vi "setHeaters.vi"(8 "error in":errorcluster, 10 "Heater2":bool, 11 "Heater1":bool) -> (0 "error out":errorcluster)   [LabVIEW 2024]
doc: "Funkcja służąca do sterowania 2 grzałkami w symulowanym piekarniku, numer wejścia odpowiada numerowi grzałki. Wartość TRUE wejścia włącza grzałkę, wartość FALSE wejścia wyłącza grzałkę."
uses:
  TypeDefs/Heater_interface.ctl
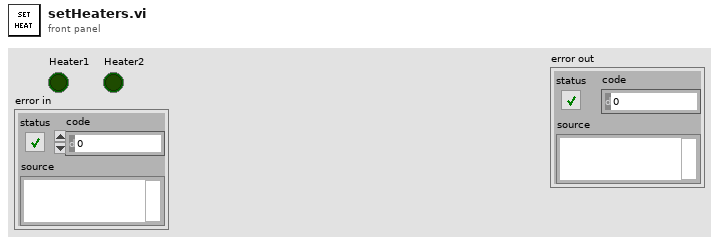
[diagram p1: front panel]
types:
  T1 = typedef "Heater_interface.ctl" = enum16{"setSpeed", "setHeaters", "getTemperature"}
  T2 = cluster{"Interface":T1, "Parameter1":variant, "Parameter2":variant}
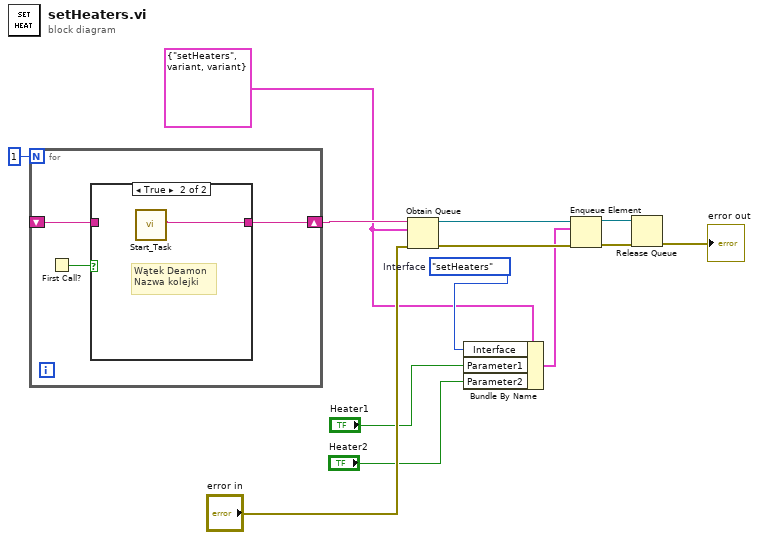
[diagram p0: block diagram]
diagram:
  w3 = T2 {"Interface"=enum."setHeaters", "Parameter1"=variant, "Parameter2"=variant}
  w4 = Heater_interface."setHeaters"  # Interface
  n1 = for {
    N: 1 -> [_]
    shift-right: [w15] -> w12
    shift-left: _ -> [w14]
    n2 = First Call?() -> (First Call?: T/F=w16:bool)
    n3 = case shown="True" w16 {
      tunnel: [w17 w18] -> w15
      tunnel: w14 -> [w17 _]
      frame False {
      }
      frame True {
        # "Wątek Deamon\nNazwa kolejki"
        n4 = call "Start_Task.vi"() -> ("QueueName"=w18:string)  [unwired: 11 in]
      }
    }
  }
  n5 = Obtain Queue(name (unnamed)=w12, element data type=w3, error in (no error)="error in") -> (queue out=w11:refnum<queue>, error out=w10:errorcluster)  [unwired: 2 in, 1 out]
  n6 = Bundle By Name(cluster=w3, "Interface"=w4, "Parameter1"="Heater1", "Parameter2"="Heater2") -> (w9:T2)
  n7 = Enqueue Element(queue=w11, element=w9, error in (no error)=w10) -> (queue out=w8:refnum<queue>, error out=w7:errorcluster)  [unwired: 1 in, 1 out]
  n8 = Release Queue(queue=w8, error in (no error)=w7) -> (error out=→"error out":errorcluster)  [unwired: 1 in, 2 out]
